vi "Case.vi"() -> ()   [LabVIEW 2020]
panel:
  out "Boolean 2":bool
  in  "Boolean":bool
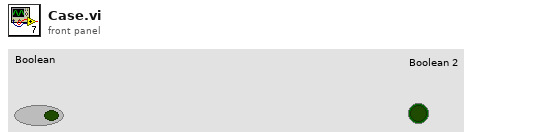
[diagram p1: front panel]
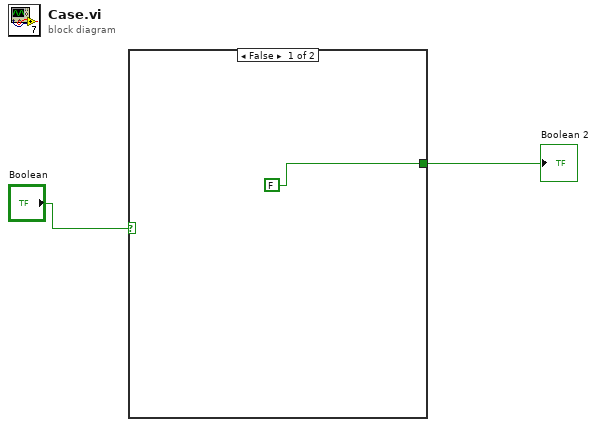
[diagram p0: block diagram]
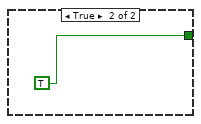
[diagram p2: hidden frame]
diagram:
  n1 = case shown="False" "Boolean" {
    tunnel: [FALSE TRUE] -> w2
    frame False {
    }
    frame True {
    }
  }
  "Boolean 2" <- w2
